vi "x-axis.vi"(8 "error in (no error)":errorcluster, 11 "Magnetic Field in":refnum<class "Magnetic Field.lvclass">) -> (0 "error out":errorcluster, 1 "Label":string, 2 "Unit":string, 3 "Magnetic Field out":refnum<class "Magnetic Field.lvclass">)   [LabVIEW 2017, in "Magnetic Field.lvclass"]
uses:
  Magnetic Field.lvclass
  Scanner/Scanner.lvclass
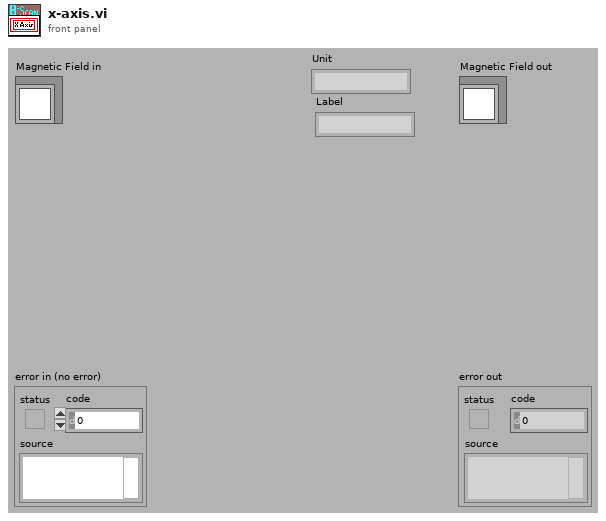
[diagram p1: front panel]
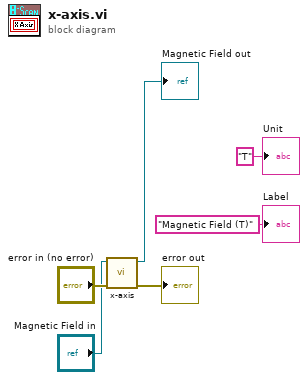
[diagram p0: block diagram]
diagram:
  n1 = call-parent "x-axis.vi"("error in (no error)"="error in (no error)", "Scanner in"="Magnetic Field in") -> ("error out"=→"error out":errorcluster, "Scanner out"=→"Magnetic Field out":refnum<class "Magnetic Field.lvclass">)  [unwired: 6 in, 2 out]
  "Label" <- "Magnetic Field (T)" ("Label")
  "Unit" <- "T" ("Unit")
